vi "Kinesis-program-one-motor-Old-Controllers.vi"() -> ()   [LabVIEW 2014]
doc: "André Romero - 2017\nandretec@ifsc.usp.br"
panel:
  out "GetPOS X":dbl=10.0 format="%^#1_6e"
  in  "GO Move":bool
  out "Motor 1":bool
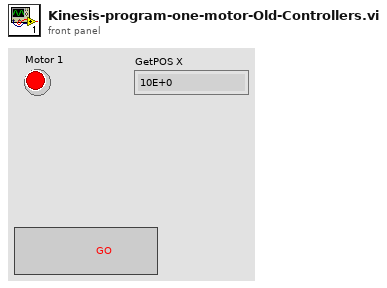
[diagram p1: front panel]
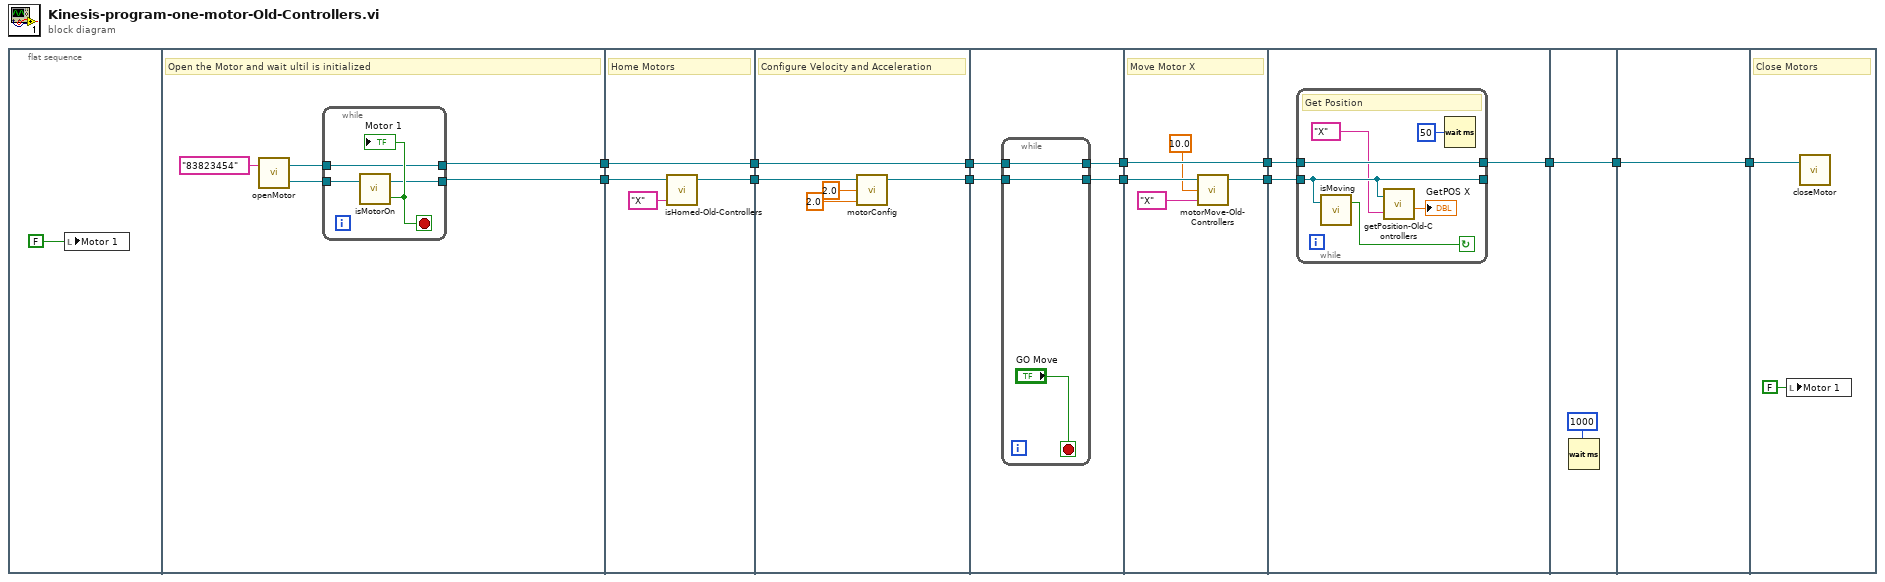
[diagram p0: block diagram]
diagram:
  n1 = flat-sequence {
    tunnel: [w19] -> w2
    tunnel: [w18] -> w1
    tunnel: w2 -> [w27]
    tunnel: w1 -> [w26]
    tunnel: [w27] -> w13
    tunnel: [w25] -> w11
    tunnel: w13 -> [w32]
    tunnel: [w32] -> w12
    tunnel: w11 -> [w28]
    tunnel: [w29] -> w10
    tunnel: w12 -> [w36]
    tunnel: [w35] -> w8
    tunnel: w10 -> [w33]
    tunnel: [w34] -> w9
    tunnel: w9 -> [w43]
    tunnel: [w42] -> w7
    tunnel: w8 -> [w44]
    tunnel: [w44] -> w6
    tunnel: w7 -> [w45]
    tunnel: w6 -> [w47]
    tunnel: [w46] -> w5
    tunnel: w5 -> [w55]
    tunnel: [w55] -> w4
    tunnel: w4 -> [w56]
    tunnel: [w56] -> w3
    tunnel: w3 -> [w58]
    frame #0 {
      n2 = local write "Motor 1"(FALSE ("isConnected")) -> ()
    }
    frame #1 {
      # "Open the Motor and wait ultil is initialized"
      n3 = call "openMotor.vi"("S/N Motor"="83823454") -> ("Device"=w16:refnum<k24>, ".NET Refnum out"=w15:refnum<k24>)  [unwired: 1 in]
      n4 = while {
        tunnel: [w22] -> w19
        tunnel: [w20] -> w18
        tunnel: w15 -> [w22]
        tunnel: w16 -> [w21]
        stop <- w23 stop-if-true
        n5 = call "isMotorOn.vi"("Device"=w21) -> ("isConnected"=w23:bool, "Device out"=w20:refnum<k24>)  [unwired: 1 in]
        "Motor 1" <- w23
      }
    }
    frame #2 {
      # "Home Motors"
      n6 = call "isHomed-Old-Controllers.vi"("Motor (XYZ)"="X", "Device in"=w26) -> ("Device out"=w25:refnum<k24>)  [unwired: 3 in]
    }
    frame #3 {
      # "Configure Velocity and Acceleration"
      n7 = call "motorConfig.vi"("Velocity"=2.0 ("MaxVelocity"), "Acceleration"=2.0, "Device in"=w28) -> ("Device out"=w29:refnum<k24>)  [unwired: 2 in]
    }
    frame #4 {
      n8 = while {
        tunnel: [w38] -> w35
        tunnel: w36 -> [w38]
        tunnel: [w37] -> w34
        tunnel: w33 -> [w37]
        stop <- "GO Move" stop-if-true
      }
    }
    frame #5 {
      # "Move Motor X"
      n9 = call "motorMove-Old-Controllers.vi"("Motor (XYZ)"="X", "position"=10.0, "Device in"=w43) -> ("Device out"=w42:refnum<k24>)  [unwired: 2 in]
    }
    frame #6 {
      n10 = while {
        tunnel: w47 -> [w53]
        tunnel: w45 -> [w50]
        tunnel: [w53] -> w46
        tunnel: [w50] -> _
        stop <- w52 continue-if-true
        # "Get Position"
        n11 = call "isMoving.vi"("Device in"=w50) -> ("IsMoving"=w52:bool)  [unwired: 1 in, 1 out]
        n12 = call "getPosition-Old-Controllers.vi"("Motor (XYZ)"="X", "Device"=w50) -> ("GetPOS"=→"GetPOS X":dbl)  [unwired: 1 in]
        n13 = Wait (ms)(milliseconds to wait=u32 50) -> ()  [unwired: 1 out]
      }
    }
    frame #7 {
      n14 = Wait (ms)(milliseconds to wait=u32 1000) -> ()  [unwired: 1 out]
    }
    frame #8 {
    }
    frame #9 {
      # "Close Motors"
      n15 = local write "Motor 1"(FALSE ("Motor 1")) -> ()
      n16 = call "closeMotor.vi"(".NET Refnum in"=w58) -> ()  [unwired: 2 in]
    }
  }
